vi "mj_mergeTerm.vi"(9 "new term":T1[](array[typedef]), 11 "old term":T1[](array[typedef])) -> (2 "merged term":T1[](array[typedef]))   [LabVIEW 2020]
uses:
  <vilib>/Platform/storage/lvStorage.llb/TerminalDef.ctl
  <vilib>/Platform/storage/lvStorage.llb/_TerminalStyle.ctl
  <vilib>/Utility/XNodeSupport.llb/XRect32.ctl
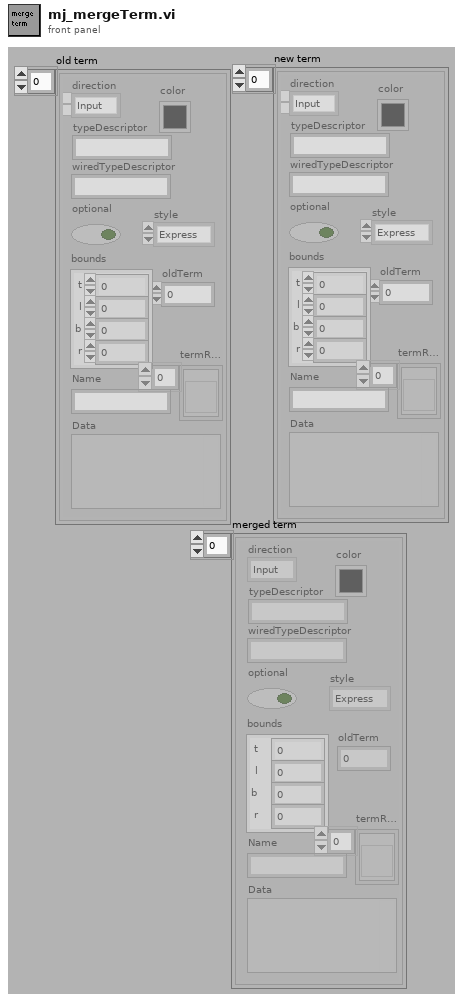
[diagram p1: front panel]
types:
  T1 = typedef "TerminalDef.ctl" = cluster{"direction":enum16{"Input", "Output"}, "typeDescriptor":string, "color":u32, "oldTerm":i32, "style":T2, "optional":bool, "bounds":T3, "termRefs":refnum<vi>[], "Name":string, "Data":variant, "wiredTypeDescriptor":string}
  T2 = typedef "_TerminalStyle.ctl" = enum16{"Express", "Collapsed", "Internal"}
  T3 = typedef "XRect32.ctl" = cluster{"t":i32, "l":i32, "b":i32, "r":i32}
  T4 = cluster{"direction":enum16{"Input", "Output"}, "Name":string}
  T5 = cluster{"direction":enum16{"Input", "Output"}, "DNL_TermID":string}
  T6 = cluster{"direction":enum16{"Input", "Output"}, "DNL_LocalizedTermName":string}
  T7 = cluster{"direction":enum16{"Input", "Output"}, "Name":string}[]
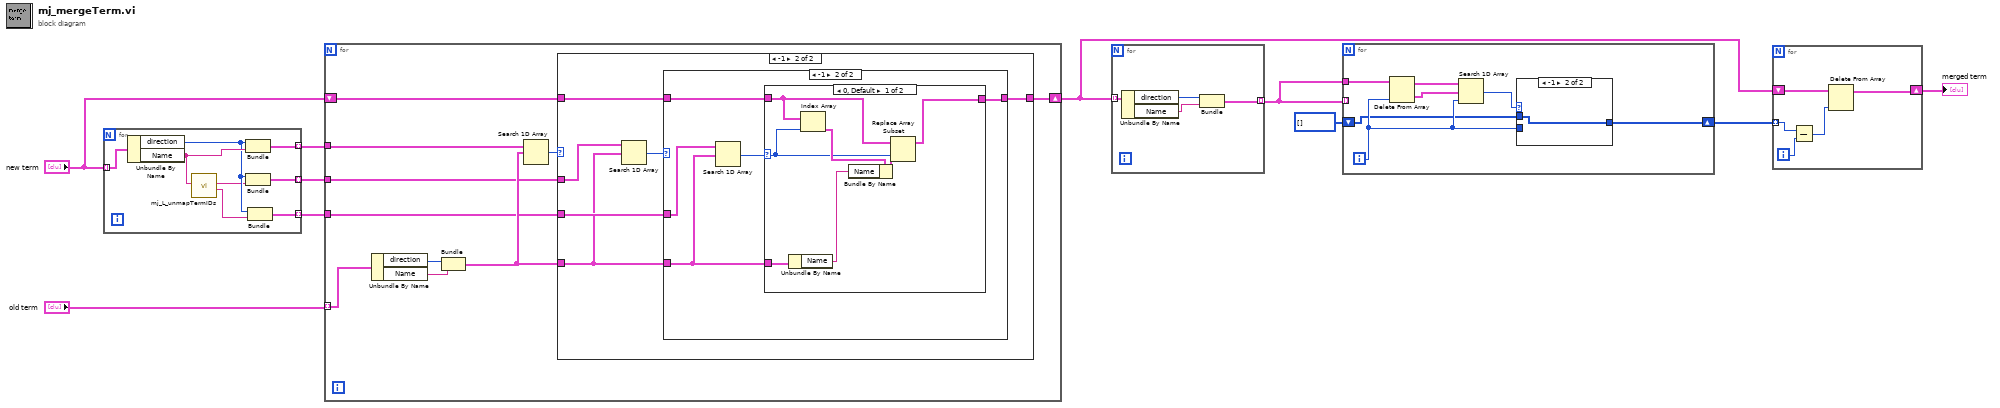
[diagram p0: block diagram]
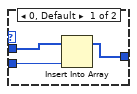
[diagram p2: hidden frame]
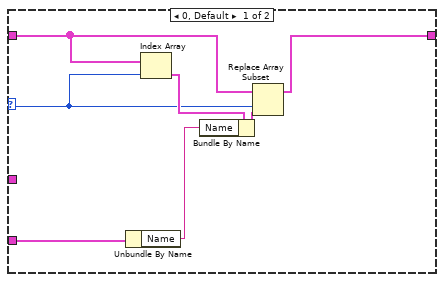
[diagram p4: hidden frame]
diagram:
  n1 = for {
    tunnel: "new term" -> [w18] mode=indexing
    tunnel: [w17] -> w10 mode=indexing
    tunnel: [w12] -> w9 mode=indexing
    tunnel: [w11] -> w8 mode=indexing
    n2 = Unbundle By Name(w18) -> ("direction"=w15:enum16{"Input", "Output"}, "Name"=w16:string)
    n3 = call <vilib>:"mj_L_unmapTermIDs.vi"("DNL_Name"=w16) -> ("DNL_LocalizedTermName"=w13:string, "DNL_TermID"=w14:string)  [unwired: 6 in, 1 out]
    n4 = Bundle("direction"=w15, "Name"=w16) -> (w17:T4)  [unwired: 1 in]
    n5 = Bundle("direction"=w15, "DNL_TermID"=w14) -> (w12:T5)  [unwired: 1 in]
    n6 = Bundle("direction"=w15, "DNL_LocalizedTermName"=w13) -> (w11:T6)  [unwired: 1 in]
  }
  n7 = for {
    tunnel: "old term" -> [w25] mode=indexing
    shift-right: [w24] -> w3
    shift-left: "new term" -> [w23]
    tunnel: w10 -> [w21]
    tunnel: w9 -> [w20]
    tunnel: w8 -> [w19]
    n8 = Unbundle By Name(w25) -> ("direction"=w28:enum16{"Input", "Output"}, "Name"=w22:string)
    n9 = Bundle("direction"=w28, "Name"=w22) -> (w26:T4)  [unwired: 1 in]
    n10 = Search 1D Array(1D array=w21, element=w26) -> (index of element=w27:i32)  [unwired: 1 in]
    n11 = case shown="-1" w27 {
      tunnel: w26 -> [_ w30]
      tunnel: [w29 w33] -> w24
      tunnel: w23 -> [w29 w34]
      tunnel: w20 -> [_ w32]
      tunnel: w19 -> [_ w31]
      frame 0, Default {
      }
      frame -1 {
        n12 = Search 1D Array(1D array=w32, element=w30) -> (index of element=w35:i32)  [unwired: 1 in]
        n13 = case shown="-1" w35 {
          selector: w35 -> [w39 _]
          tunnel: w34 -> [w38 w47]
          tunnel: [w37 w46] -> w33
          tunnel: w31 -> [_ w44]
          tunnel: w30 -> [w36 w43]
          frame 0, Default {
            n14 = Unbundle By Name(w36) -> ("Name"=w40:string)
            n15 = Index Array(array=w38, index=w39) -> (element=w42:T1)
            n16 = Bundle By Name(cluster=w42, "Name"=w40) -> (w41:T1)
            n17 = Replace Array Subset(array=w38, new element=w41, index=w39) -> (w37:T1[])
          }
          frame -1 {
            n18 = Search 1D Array(1D array=w44, element=w43) -> (index of element=w45:i32)  [unwired: 1 in]
            n19 = case shown="0, Default" w45 {
              selector: w45 -> [w50 _]
              tunnel: w47 -> [w54 w55]
              tunnel: [w53 w55] -> w46
              tunnel: w43 -> [w52 _]
              frame 0, Default {
                n20 = Unbundle By Name(w52) -> ("Name"=w48:string)
                n21 = Index Array(array=w54, index=w50) -> (element=w51:T1)
                n22 = Bundle By Name(cluster=w51, "Name"=w48) -> (w49:T1)
                n23 = Replace Array Subset(array=w54, new element=w49, index=w50) -> (w53:T1[])
              }
              frame -1 {
              }
            }
          }
        }
      }
    }
  }
  n24 = for {
    tunnel: w3 -> [w59] mode=indexing
    tunnel: [w56] -> w5 mode=indexing
    n25 = Unbundle By Name(w59) -> ("direction"=w58:enum16{"Input", "Output"}, "Name"=w57:string)
    n26 = Bundle("direction"=w58, "Name"=w57) -> (w56:T4)  [unwired: 1 in]
  }
  n27 = for {
    tunnel: w5 -> [_] mode=indexing
    tunnel: w5 -> [w66]
    shift-right: [w61] -> w2
    shift-left: i32[] [] -> [w60]
    i -> [w62]
    n28 = Delete From Array(array=w66, index=w62) -> (deleted portion=w65:T4, array with subset deleted=w64:T7)  [unwired: 1 in]
    n29 = Search 1D Array(1D array=w64, element=w65, start index (0)=w62) -> (index of element=w63:i32)
    n30 = case shown="-1" w63 {
      tunnel: w62 -> [w69 _]
      tunnel: [w68 w70] -> w61
      tunnel: w60 -> [w67 w70]
      frame 0, Default {
        n31 = Insert Into Array(array=w67, new element=w69) -> (w68:i32[])  [unwired: 1 in]
      }
      frame -1 {
      }
    }
  }
  n32 = for {
    shift-right: [w71] -> w1
    shift-left: w3 -> [w75]
    tunnel: w2 -> [w74] mode=indexing
    i -> [w73]
    n33 = Subtract(x=w74, y=w73) -> (x-y=w72:i32)
    n34 = Delete From Array(array=w75, index=w72) -> (array with subset deleted=w71:T1[])  [unwired: 1 in, 1 out]
  }
  "merged term" <- w1
